vi "下载文件.vi"(1 "URL":string) -> (0 "下载成功?":bool=TRUE)   [LabVIEW 2018]
uses:
  <vilib>/AppBuilder/AB_API_Simple/NI_App_Builder_API.lvlib
  <vilib>/AppBuilder/AB_API_Simple/Get Build Specification Version (path).vi
panel:
  out "数值 4":i32
  out "数值 3":i32
  out "数值 2":i32
  out "数值":i32
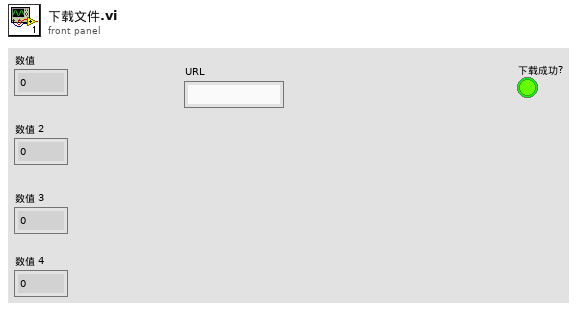
[diagram p1: front panel]
types:
  T1 = typedef "NI_App_Builder_API.lvlib/Build Specification Version.ctl" = cluster{"Major":u16, "Minor":u16, "Fix":u16, "Build":u16}
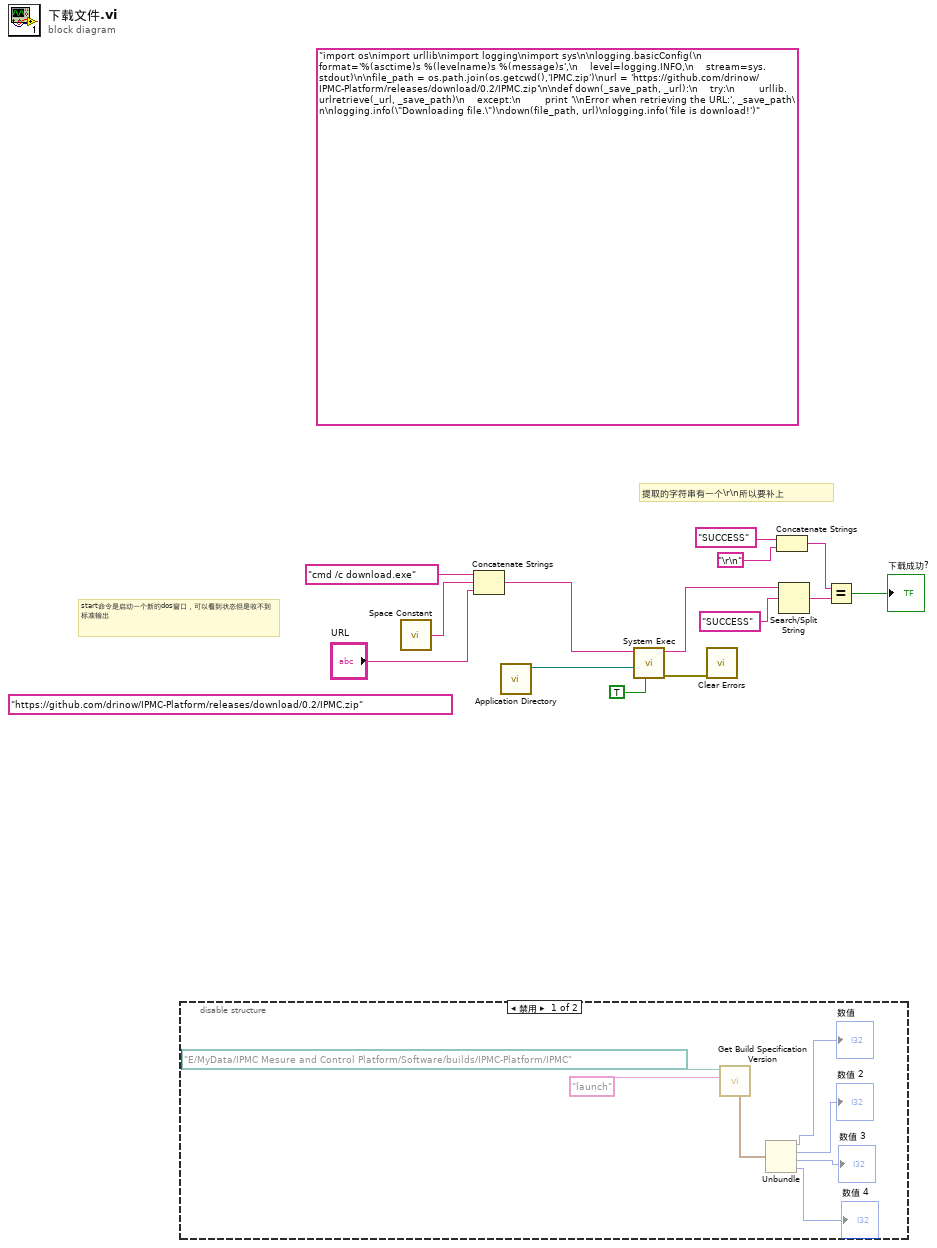
[diagram p0: block diagram]
diagram:
  (unwired) "https://github.com/drinow/IPMC-Platform/releases/download/0.2/IPMC.zip"
  (unwired) "import os\nimport urllib\nimport logging\nimport sys\n\nlogging.basicConfig(\n    format='%(asctime)s %(levelname)s %(message)s',\n    level=logging.INFO,\n    stream=sys.stdout)\n\nfile_path = os.path.join(os.getcwd(),'IPMC.zip')\nurl = 'https://github.com/drinow/IPMC-Platform/releases/download/0.2/IPMC.zip'\n\ndef down(_save_path, _url):\n    try:\n        urllib.urlretrieve(_url, _save_path)\n    except:\n        print '\\nError when retrieving the URL:', _save_path\n\nlogging.info(\"Downloading file.\")\ndown(file_path, url)\nlogging.info('file is download!')"
  # "提取的字符串有一个\\r\\n所以要补上"
  # "start命令是启动一个新的dos窗口，可以看到状态但是收不到标准输出"
  n1 = disable-structure shown="禁用" {
    frame Disabled {
      n2 = call-poly <vilib>:"Get Build Specification Version.vi"("Name of build specification"="launch", "Path to project"=path "E:/MyData/IPMC Mesure and Control Platform/Software/builds/IPMC-Platform/IPMC") -> ("Build Specification Version"=w19:T1)  [unwired: 8 in, 1 out]
      n3 = Unbundle(w19) -> ("Major"=→"数值":u16, "Minor"=→"数值 2":u16, "Fix"=→"数值 3":u16, "Build"=→"数值 4":u16)
    }
    frame Enabled {
    }
  }
  n4 = call <vilib>:"Space Constant.vi"() -> ("String"=w6:string)
  n5 = Concatenate Strings("cmd /c download.exe", w6, "URL") -> (w5:string)
  n6 = call <vilib>:"Application Directory.vi"() -> ("Application Directory"=w13:path)
  n7 = call <vilib>:"System Exec.vi"("run minimized? (F)"=TRUE, "working directory"=w13, "command line"=w5) -> ("error out"=w12:errorcluster, "standard output"=w10:string)  [unwired: 5 in, 2 out]
  n8 = call <vilib>:"Clear Errors.vi"("error in (no error)"=w12) -> ()  [unwired: 5 in, 2 out]
  n9 = Concatenate Strings("SUCCESS", "\r\n") -> (w2:string)
  n10 = Search/Split String(string=w10, search string/char (-)="SUCCESS") -> (match + rest of string=w9:string)  [unwired: 1 in, 2 out]
  n11 = Equal?(x=w2, y=w9) -> (x = y?=→"下载成功?":bool)
